vi "preAmplifier.vi"(11 "Pre Code":u8) -> ()   [LabVIEW 2009]
doc: "Receives a Byte with the Gain Information for both the A and B Pre-amplifiers and sets the amplifiers accordingly. B is sent first beginning by the MSB."
uses:
  <vilib>/eio/EIONode/EIONode.xnode
  <vilib>/rvi/eio/nirviEIOImplementation/nirviEIOImplementation.xnode
  <vilib>/rvi/eio/common/nirviEmuTemplateMethod_noerrors.vi
  <vilib>/rvi/eio/common/nirviEmuClasses.ctl
  Instance           4 20Saved   preAmplifier .vi
  Instance           3 20Saved   preAmplifier .vi
  Instance           2 20Saved   preAmplifier .vi
  Instance           1 20Saved   preAmplifier .vi
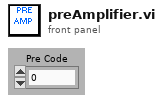
[diagram p1: front panel]
types:
  T1 = typedef "nirviEmuClasses.ctl" = enum16{"IO Read", "IO Write", "Method", "Property Read", "Property Write"}
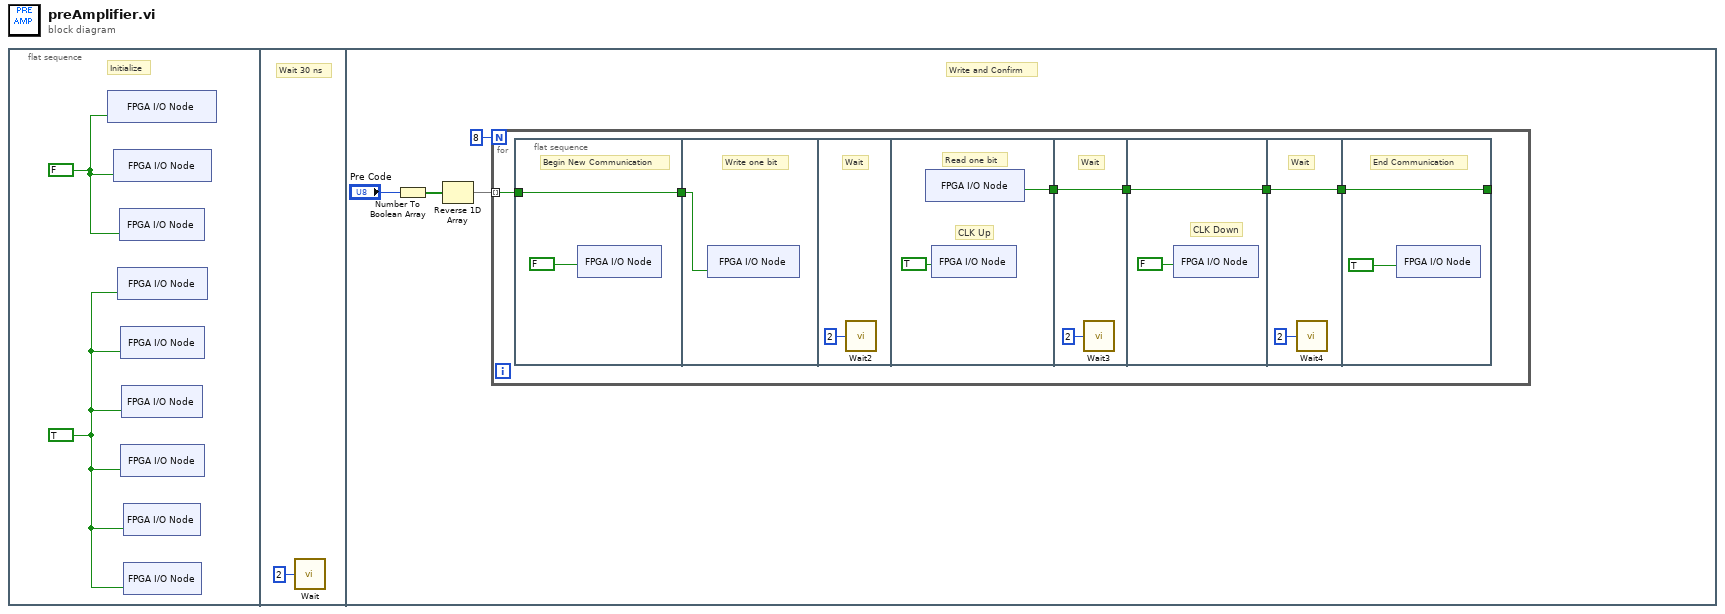
[diagram p0: block diagram]
diagram:
  n1 = flat-sequence {
    frame #0 {
      w2 = TRUE
      w1 = FALSE ("AMP_SHDN")
      # "Initialize"
      n2 = xnode "FPGA I/O Node"("FPGA_INIT_B"=w1) -> ()  [unwired: 1 in, 1 out]
      n3 = xnode "FPGA I/O Node"("AMP_SHDN"=w1) -> ()  [unwired: 1 in, 1 out]
      n4 = xnode "FPGA I/O Node"("SPI_SS_B"=w2) -> ()  [unwired: 1 in, 1 out]
      n5 = xnode "FPGA I/O Node"("SPI_SCK"=w1) -> ()  [unwired: 1 in, 1 out]
      n6 = xnode "FPGA I/O Node"("AMP_CS"=w2) -> ()  [unwired: 1 in, 1 out]
      n7 = xnode "FPGA I/O Node"("DAC_CS"=w2) -> ()  [unwired: 1 in, 1 out]
      n8 = xnode "FPGA I/O Node"("SF_CE0"=w2) -> ()  [unwired: 1 in, 1 out]
      n9 = xnode "FPGA I/O Node"("SF_OE"=w2) -> ()  [unwired: 1 in, 1 out]
      n10 = xnode "FPGA I/O Node"("SF_WE"=w2) -> ()  [unwired: 1 in, 1 out]
    }
    frame #1 {
      # "Wait 30 ns"
      n11 = call "Wait"("Count(Ticks)"=u32 2) -> ()  [unwired: 1 out]
    }
    frame #2 {
      # "Write and Confirm"
      n12 = Number To Boolean Array(number="Pre Code") -> (Boolean array=w112:bool[])
      n13 = Reverse 1D Array(array=w112) -> (reversed array=w113:bool[])
      n14 = for {
        N: 8 -> [_]
        tunnel: w113 -> [w121] mode=indexing
        n15 = flat-sequence {
          tunnel: w121 -> [w122]
          tunnel: [w122] -> w117
          tunnel: w117 -> [w136]
          tunnel: [w150] -> w118
          tunnel: [w184] -> w119
          tunnel: w118 -> [w184]
          tunnel: [w186] -> w120
          tunnel: w119 -> [w186]
          tunnel: w120 -> [w201]
          tunnel: [w201] -> w116
          tunnel: [w203] -> _
          tunnel: w116 -> [w203]
          frame #0 {
            # "Begin New Communication"
            n16 = xnode "FPGA I/O Node"("AMP_CS"=FALSE) -> ()  [unwired: 1 in, 1 out]
          }
          frame #1 {
            # "Write one bit"
            n17 = xnode "FPGA I/O Node"("SPI_MOSI"=w136) -> ()  [unwired: 1 in, 1 out]
          }
          frame #2 {
            # "Wait"
            n18 = call "Wait2"("Count(Ticks)"=u32 2) -> ()  [unwired: 1 out]
          }
          frame #3 {
            # "CLK Up"
            # "Read one bit"
            n19 = xnode "FPGA I/O Node"() -> ("AMP_DOUT"=w150:bool)  [unwired: 1 in, 1 out]
            n20 = xnode "FPGA I/O Node"("SPI_SCK"=TRUE) -> ()  [unwired: 1 in, 1 out]
          }
          frame #4 {
            # "Wait"
            n21 = call "Wait3"("Count(Ticks)"=u32 2) -> ()  [unwired: 1 out]
          }
          frame #5 {
            # "CLK Down"
            n22 = xnode "FPGA I/O Node"("SPI_SCK"=FALSE) -> ()  [unwired: 1 in, 1 out]
          }
          frame #6 {
            # "Wait"
            n23 = call "Wait4"("Count(Ticks)"=u32 2) -> ()  [unwired: 1 out]
          }
          frame #7 {
            # "End Communication"
            n24 = xnode "FPGA I/O Node"("AMP_CS"=TRUE) -> ()  [unwired: 1 in, 1 out]
          }
        }
      }
    }
  }
